vi "send_step.vi"(2 "error in":errorcluster, 3 "message":string="{\"amount\":1}", 4 "Command_ID":string="REPLAY_StepSimulationCommand_ID") -> (0 "error out":errorcluster)   [LabVIEW 2019, in "Lib_Simx.lvlib"]
doc: "Send the command to step the simulation for any given amount. Specify the desired amount in the message string."
uses:
  Lib_Simx.lvlib
  tools/simx_common.vi
panel:
  out "success":bool
  out "config response":string
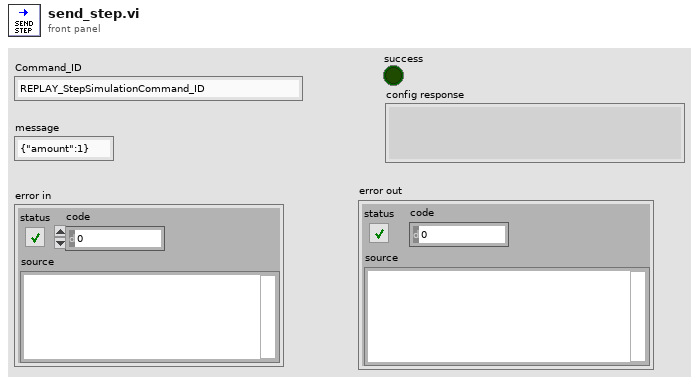
[diagram p1: front panel]
types:
  T1 = typedef "Lib_Simx.lvlib/simx_connection.ctl" = cluster{"Config":T2, "Connections":T5, "Map":cluster{"lanes":cluster{"x":dbl[], "y":dbl[], "z":dbl[]}, "StartPosition":cluster{"start_points":T6, "StartRotation":dbl[], "StartLocation":dbl[]}, "Draw Map Size":T7, "DrawArea":cluster{"min_Y":dbl, "min_X":dbl, "Scale X":dbl, "Scale Y":dbl}, "Map":picture, "Map Geojson":string}}
  T2 = typedef "Lib_Simx.lvlib/config.ctl" = cluster{"Trajectory":T3, "Weather":T4}
  T3 = typedef "Lib_Simx.lvlib/trajectory.ctl" = cluster{"Number of frames":i32, "Frame number":i32, "Trajectory":string}
  T4 = typedef "Lib_Simx.lvlib/weather.ctl" = cluster{"id":string}
  T5 = typedef "Lib_Simx.lvlib/connections.ctl" = cluster{"Simulator Connection":refnum<k5>, "server_ip":string, "Port":i32, "Sensor connections":refnum<k5>[]}
  T6 = typedef "Lib_Simx.lvlib/start_points.ctl" = cluster{"locations":dbl[][], "rotations":dbl[][], "type":string[]}
  T7 = typedef "LVBoundsTypeDef.ctl" = cluster{"Width":u32, "Height":u32}
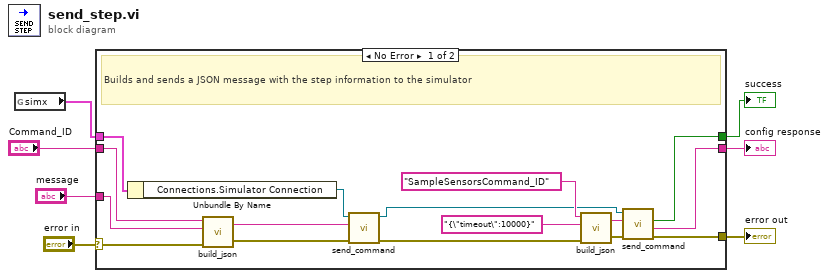
[diagram p0: block diagram]
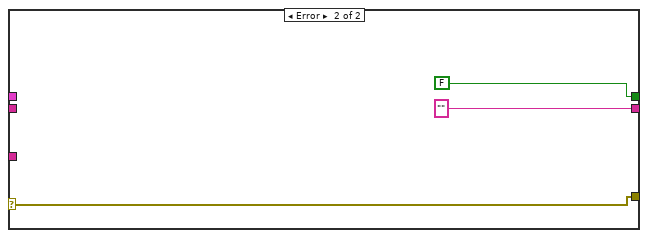
[diagram p2: hidden frame]
diagram:
  n1 = global read "simx_common.vi" "simx"() -> (w1:T1)
  n2 = case shown="No Error" "error in" {
    selector: "error in" -> [w23 w26]
    tunnel: [w13 w26] -> w7
    tunnel: "message" -> [w20 _]
    tunnel: "Command_ID" -> [w22 _]
    tunnel: [w10 "" ("response")] -> w3
    tunnel: [w9 FALSE ("success")] -> w2
    tunnel: w1 -> [w21 _]
    frame No Error {
      # "Builds and sends a JSON message with the step information to the simulator"
      n3 = Unbundle By Name(w21) -> ("Connections.Simulator Connection"=w18:refnum<k5>)
      n4 = call "build_json.vi"("error in"=w23, "Message"=w20, "Command_ID"=w22) -> ("error out"=w19:errorcluster, "JSON Out"=w17:string)  [unwired: 1 in]
      n5 = call "send_command.vi"("error in"=w19, "JSON Command"=w17, "TCP Network Connection in"=w18) -> ("error out"=w14:errorcluster, "TCP Network Connection Out"=w8:refnum<k5>)  [unwired: 1 in, 2 out]
      n6 = call "build_json.vi"("error in"=w14, "Message"="{\"timeout\":10000}", "Command_ID"="SampleSensorsCommand_ID") -> ("error out"=w15:errorcluster, "JSON Out"=w16:string)  [unwired: 1 in]
      n7 = call "send_command.vi"("error in"=w15, "JSON Command"=w16, "TCP Network Connection in"=w8) -> ("error out"=w13:errorcluster, "Response"=w10:string, "Success"=w9:bool)  [unwired: 1 in, 1 out]
    }
    frame Error {
    }
  }
  "error out" <- w7
  "config response" <- w3
  "success" <- w2
